vi "test CompactSubObj.vi"(11 "Test Case In":refnum<class "Test EDS.lvclass">) -> (0 "error out":errorcluster, 3 "Test Case Out":refnum<class "Test EDS.lvclass">)   [LabVIEW 2024, in "Test EDS.lvclass"]
uses:
  Test EDS.lvclass
  Test EDS.lvclass/Test EDS.ctl
  4993e8ee-a06a-463a-9684-69129f64d5ce.vi
  Core/EDS/EDS.lvclass
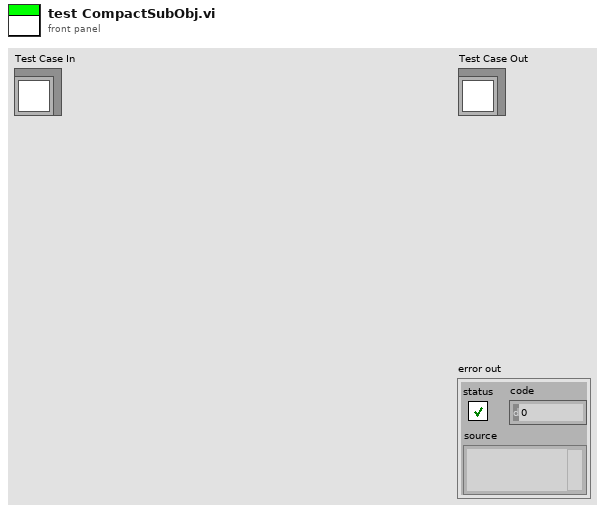
[diagram p1: front panel]
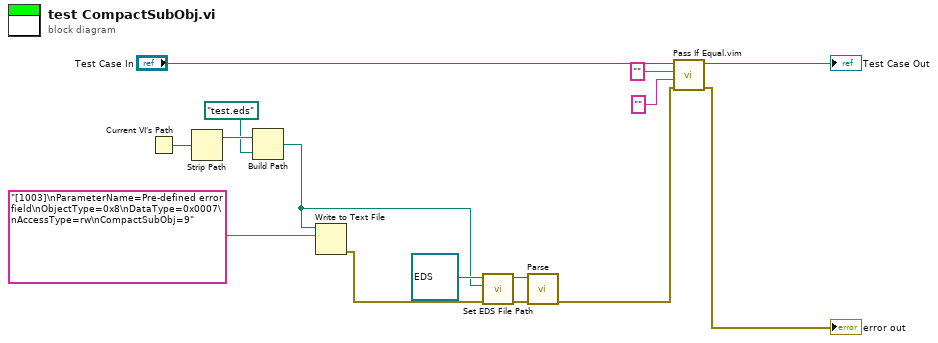
[diagram p0: block diagram]
diagram:
  n1 = Current VI's Path() -> (path=w8:path)
  n2 = Strip Path(path=w8) -> (stripped path=w7:path)  [unwired: 1 out]
  n3 = Build Path(base path=w7, name or relative path=path "test.eds") -> (appended path=w2:path)
  n4 = Write to Text File(file (use dialog)=w2, text="[1003]\nParameterName=Pre-defined error field\nObjectType=0x8\nDataType=0x0007\nAccessType=rw\nCompactSubObj=9") -> (error out=w5:errorcluster)  [unwired: 2 in, 2 out]
  n5 = call "Set EDS File Path.vi"("EDS File Path"=w2, "EDS in"=refnum<class "EDS.lvclass"> refnum ("EDS.lvlib:EDS.lvclass")) -> ("EDS out"=w3:refnum<class "EDS.lvclass">)  [unwired: 9 in]
  n6 = call "Parse.vi"("error in"=w5, "EDS in"=w3) -> ("error out"=w10:errorcluster)  [unwired: 8 in, 1 out]
  n7 = call "Pass If Equal.vim"("error in (no error)"=w10, "Actual"="", "Expected"="", "LUnit Test Case In"="Test Case In") -> ("error out"=→"error out":errorcluster, "LUnit Test Case Out"=→"Test Case Out":refnum<class "Test EDS.lvclass">)  [unwired: 6 in]
